vi "DROPBEAR_Model_Updating_FEA_KF.vi"(8 "error in (no error)":errorcluster, 11 "DROPBEAR_Model_Updating in":refnum<class "DROPBEAR_Model_Updating.lvclass">) -> (0 "error out":errorcluster, 3 "DROPBEAR_Model_Updating out":refnum<class "DROPBEAR_Model_Updating.lvclass">)   [LabVIEW 2021, in "DROPBEAR_Model_Updating.lvclass"]
uses:
  DROPBEAR_Model_Updating.lvclass
  DROPBEAR_Model_Updating.lvclass/DROPBEAR_Model_Updating.ctl
  Kalman_Filter/Kalman_Filter.lvclass
  FEA_Model/FEA_Model.lvclass
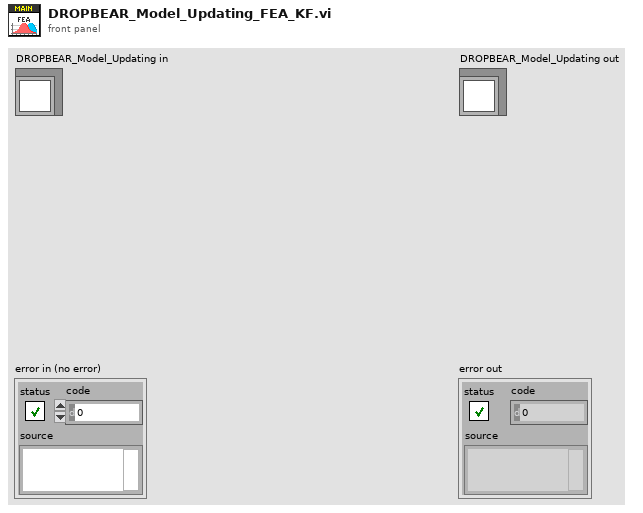
[diagram p1: front panel]
types:
  T1 = enum16{"Scalar Particle to Meter", "Scalar Node to Meter", "Scalar Meter to Particle", "Scalar Meter to Node", "Array Particle to Meter", "Array Node to Meter", "Array Meter to Particle", "Array Meter to Node"}
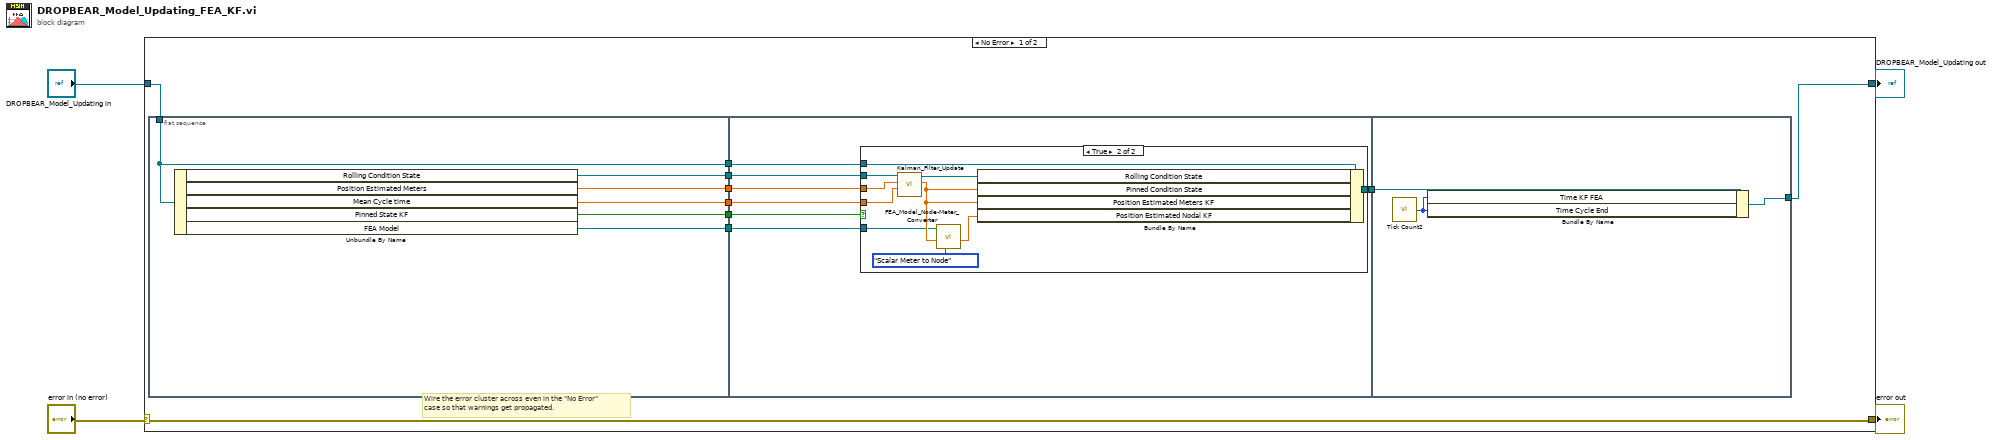
[diagram p0: block diagram]
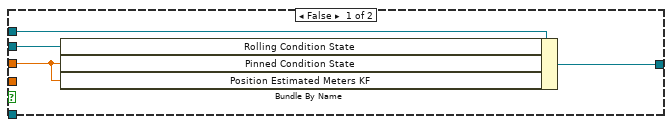
[diagram p2: hidden frame]
diagram:
  n1 = case shown="No Error" "error in (no error)" {
    selector: "error in (no error)" -> [w14 w46]
    tunnel: [w14 w46] -> w3
    tunnel: [w6 w45] -> w1
    tunnel: "DROPBEAR_Model_Updating in" -> [w13 w45]
    frame No Error {
      # "Wire the error cluster across even in the \"No Error\"\ncase so that warnings get propagated."
      n2 = flat-sequence {
        tunnel: w13 -> [w18]
        tunnel: [w20] -> w12
        tunnel: [w19] -> w11
        tunnel: [w16] -> w10
        tunnel: [w18] -> w9
        tunnel: [w17] -> w8
        tunnel: [w15] -> w5
        tunnel: w12 -> [w27]
        tunnel: w11 -> [w26]
        tunnel: w10 -> [w25]
        tunnel: w9 -> [w24]
        tunnel: w8 -> [w23]
        tunnel: [w22] -> w7
        tunnel: w5 -> [w21]
        tunnel: w7 -> [w44]
        tunnel: [w43] -> w6
        frame #0 {
          n3 = Unbundle By Name(w18) -> ("Rolling Condition State"=w20:refnum<class "Kalman_Filter.lvclass">, "Position Estimated Meters"=w19:dbl, "Mean Cycle time"=w16:dbl, "Pinned State KF"=w17:bool, "FEA Model"=w15:refnum<class "FEA_Model.lvclass">)
        }
        frame #1 {
          n4 = case shown="True" w23 {
            tunnel: w27 -> [w30 w41]
            tunnel: w26 -> [w31 w37]
            tunnel: w25 -> [_ w36]
            tunnel: w24 -> [w29 w40]
            tunnel: [w28 w38] -> w22
            tunnel: w21 -> [_ w32]
            frame False {
              n5 = Bundle By Name(cluster=w29, "Rolling Condition State"=w30, "Pinned Condition State"=w31, "Position Estimated Meters KF"=w31) -> (w28:refnum<class "DROPBEAR_Model_Updating.lvclass">)
            }
            frame True {
              n6 = call "Kalman_Filter_Update.vi"("T Sample"=w36, "New Measurement"=w37, "Kalman_Filter in"=w41) -> ("Estimate"=w35:dbl, "Kalman_Filter out"=w39:refnum<class "Kalman_Filter.lvclass">)  [unwired: 6 in, 1 out]
              n7 = call "FEA_Model_Node-Meter_Converter.vi"("Conversion Mode"=T1."Scalar Meter to Node", "Scalar in"=w35, "FEA_Model in"=w32) -> ("Scalar out"=w33:dbl)  [unwired: 5 in, 3 out]
              n8 = Bundle By Name(cluster=w40, "Rolling Condition State"=w39, "Pinned Condition State"=w35, "Position Estimated Meters KF"=w35, "Position Estimated Nodal KF"=w33) -> (w38:refnum<class "DROPBEAR_Model_Updating.lvclass">)
            }
          }
        }
        frame #2 {
          n9 = call "Tick Count2"() -> ("Tick Count(uSec)"=w42:u32)
          n10 = Bundle By Name(cluster=w44, "Time KF FEA"=w42, "Time Cycle End"=w42) -> (w43:refnum<class "DROPBEAR_Model_Updating.lvclass">)
        }
      }
    }
    frame Error {
    }
  }
  "error out" <- w3
  "DROPBEAR_Model_Updating out" <- w1
